vi "Get Steering Wheel Parameters.vi"(8 "error in (no error)":errorcluster, 11 "steering wheel in":refnum<class "NI_Robotics_Steering Wheel.lvclass">) -> (0 "error out":errorcluster, 2 "steering parameters":T1={"steering gear ratio"=1.0, "motor angle offset (rad)"=0.0, "steering angle range"={"min steering angle (rad)"=-3.14159, "max steering angle (rad)"=3.141592653589793}}, 3 "steering wheel out":refnum<class "NI_Robotics_Steering Wheel.lvclass">)   [LabVIEW 2017, in "NI_Robotics_Steering Wheel.lvclass"]
uses:
  <vilib>/robotics/Steering/Steering Wheel/NI_Robotics_Steering Wheel.lvclass
  <vilib>/robotics/Steering/Steering Wheel/Steering Wheel Parameters.ctl
  <vilib>/robotics/Steering/Steering Wheel/Steering Angle Range.ctl
  <vilib>/robotics/Steering/Steering Wheel/NI_Robotics_Steering Wheel.lvclass/NI_Robotics_Steering Wheel.ctl
  <vilib>/Analysis/coordinate.llb/Wrap Angle (scalar).vi
  <vilib>/Analysis/NI_AAL_Angle.lvlib
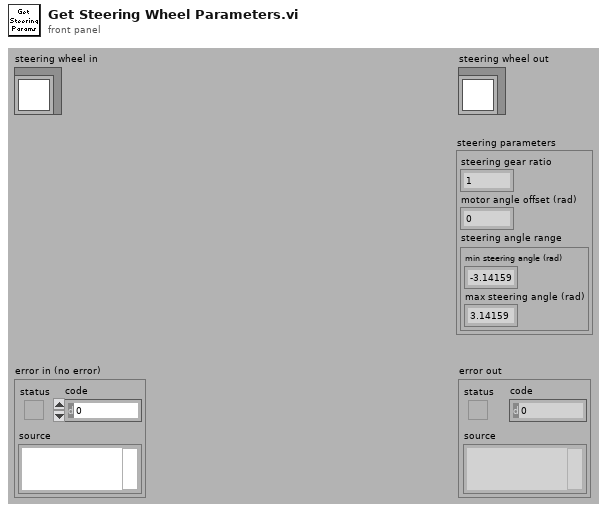
[diagram p1: front panel]
types:
  T1 = typedef "NI_Robotics_Steering Wheel.lvclass/Steering Wheel Parameters.ctl" = cluster{"steering gear ratio":dbl, "motor angle offset (rad)":dbl, "steering angle range":T2}
  T2 = typedef "NI_Robotics_Steering Wheel.lvclass/Steering Angle Range.ctl" = cluster{"min steering angle (rad)":dbl, "max steering angle (rad)":dbl}
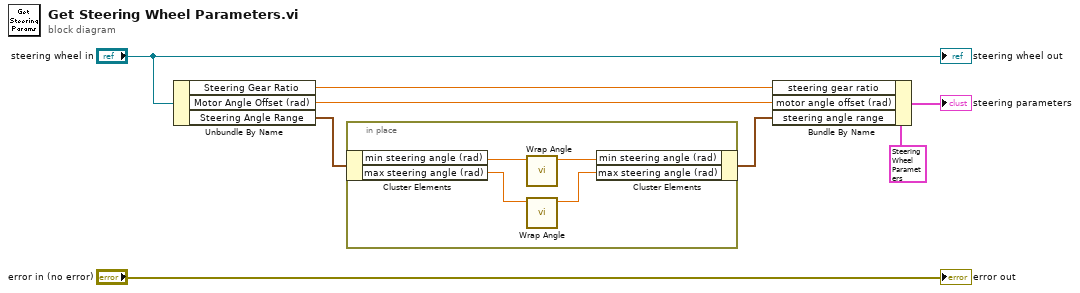
[diagram p0: block diagram]
diagram:
  n1 = Unbundle By Name("steering wheel in") -> ("Steering Gear Ratio"=w6:dbl, "Motor Angle Offset (rad)"=w5:dbl, "Steering Angle Range"=w2:T2)
  n2 = in-place {
    n3 = in-place-cluster #1(w2) -> ("min steering angle (rad)"=w12:dbl, "max steering angle (rad)"=w10:dbl)
    n4 = call-poly <vilib>:"Wrap Angle.vi"("angle in"=w12) -> ("angle out"=w11:dbl)  [unwired: 9 in, 1 out]
    n5 = call-poly <vilib>:"Wrap Angle.vi"("angle in"=w10) -> ("angle out"=w9:dbl)  [unwired: 9 in, 1 out]
    n6 = in-place-cluster #1("min steering angle (rad)"=w11, "max steering angle (rad)"=w9) -> (w1:T2)
  }
  n7 = Bundle By Name(cluster=T1 {"steering gear ratio"=1.0, "motor angle offset (rad)"=0.0, "steering angle range"={"min steering angle (rad)"=-3.14159, "max steering angle (rad)"=3.141592653589793}} ("steering wheel parameters"), "steering gear ratio"=w6, "motor angle offset (rad)"=w5, "steering angle range"=w1) -> (→"steering parameters":T1)
  "error out" <- "error in (no error)"
  "steering wheel out" <- "steering wheel in"
